vi "write default value Array of U16.vi"(8 "error in":errorcluster, 10 "default value":u16[](array[numeric]), 11 "system tag in":refnum<class "tag descriptor.lvclass">) -> (0 "error out":errorcluster, 3 "system tag out":refnum<class "tag descriptor.lvclass">)   [LabVIEW 2013, in "tag bus.lvlib" / "tag descriptor.lvclass"]
doc: "Converts the provided default value into a string and stores that as the raw default value within the tag."
uses:
  tag descriptor.lvclass
  Data Type.ctl
  tag descriptor.lvclass/tag descriptor.ctl
  tag bus.lvlib
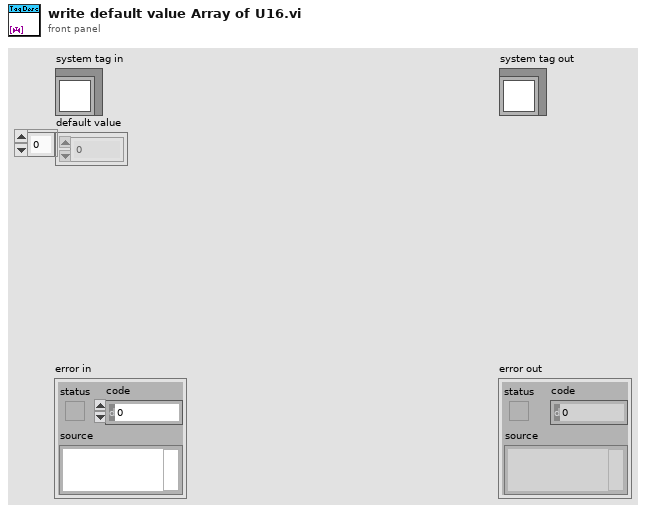
[diagram p1: front panel]
types:
  T1 = typedef "tag bus.lvlib/tag descriptor.lvclass/Data Type.ctl" = enum16{"Double", "Single", "I64", "I32", "I16", "I8", "U64", "U32", "U16", "U8", "Boolean", "String", "Array of Double", "Array of Single", "Array of I64", "Array of I32", "Array of I16", "Array of I8", "Array of U64", "Array of U32", "Array of U16", "Array of U8", "Array of Boolean", "Array of String"}
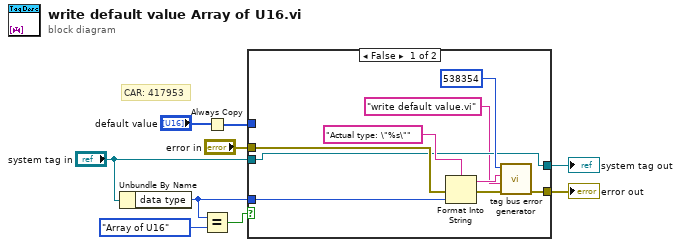
[diagram p0: block diagram]
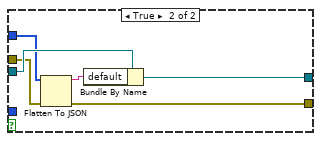
[diagram p2: hidden frame]
diagram:
  # "CAR: 417953"
  n1 = Unbundle By Name("system tag in") -> ("data type"=w5:T1)
  n2 = Always Copy(1:"default value") -> (0:w1:u16[])
  n3 = Equal?(x=w5, y=Data_Type."Array of U16") -> (x = y?=w8:bool)
  n4 = case shown="False" w8 {
    tunnel: "error in" -> [w18 w22]
    tunnel: [w14 w19] -> w6
    tunnel: w5 -> [w13 _]
    tunnel: [w11 w23] -> w4
    tunnel: "system tag in" -> [w11 w24]
    tunnel: w1 -> [_ w21]
    frame False {
      n5 = Format Into String(format string="Actual type: \"%s\"", error in=w18, w13) -> (resulting string=w15:string, error out=w16:errorcluster)  [unwired: 1 in]
      n6 = call "tag bus error generator.vi"("error in"=w16, "source"="write default value.vi", "append error message"=w15, "error code (0)"=538354) -> ("error out"=w14:errorcluster)  [unwired: 5 in]
    }
    frame True {
      n7 = Flatten To JSON(anything=w21, error in (no error)=w22) -> (JSON string=w20:string, 11:w19:errorcluster)  [unwired: 1 in]
      n8 = Bundle By Name(cluster=w24, "default"=w20) -> (w23:refnum<class "tag descriptor.lvclass">)
    }
  }
  "error out" <- w6
  "system tag out" <- w4
